vi "Read SVID File.vi"(8 "error in":errorcluster) -> (0 "error out":errorcluster, 3 "SVID Data":T1[](array[typedef]))   [LabVIEW 2020, in "SECS Communication.lvlib" / "SECS Data Class.lvclass"]
uses:
  SECS Data Class.lvclass
  SVID Data.ctl
  SECS-II Class/Format Code.ctl
  <vilib>/DATA AHEAD/XLR8/functions/Workbook/Open Create Workbook XLSX.vi
  <vilib>/DATA AHEAD/XLR8/XLR8.lvlib
  SECS-II Class/SECS-II Class.lvclass
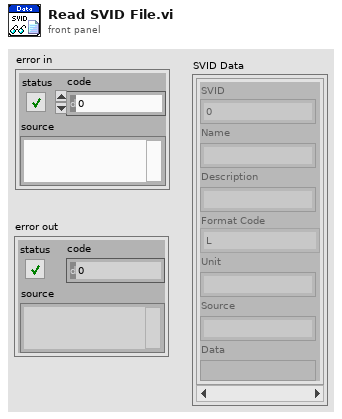
[diagram p1: front panel]
types:
  T1 = typedef "SECS Communication.lvlib/SECS Data Class.lvclass/SVID Data.ctl" = cluster{"SVID":u32, "Name":string, "Description":string, "Format Code":T2, "Unit":string, "Source":string, "Data":variant}
  T2 = typedef "SECS Communication.lvlib/SECS-II Class.lvclass/Format Code.ctl" = enum16{"L", "A", "B", "Boolean", "J", "I1", "I2", "I4", "I8", "U1", "U2", "U4", "U8", "F4", "F8", "Char"}
  T3 = typedef "XLR8.lvlib/XLR8_Ref.ctl" = cluster{"WBK":refnum<k24>, "CurSheet":refnum<k24>, "File":refnum<k24>, "file path":string, "sheet":string, "Sheets":refnum<k24>[], "IsXML":bool, "Policy":i32}
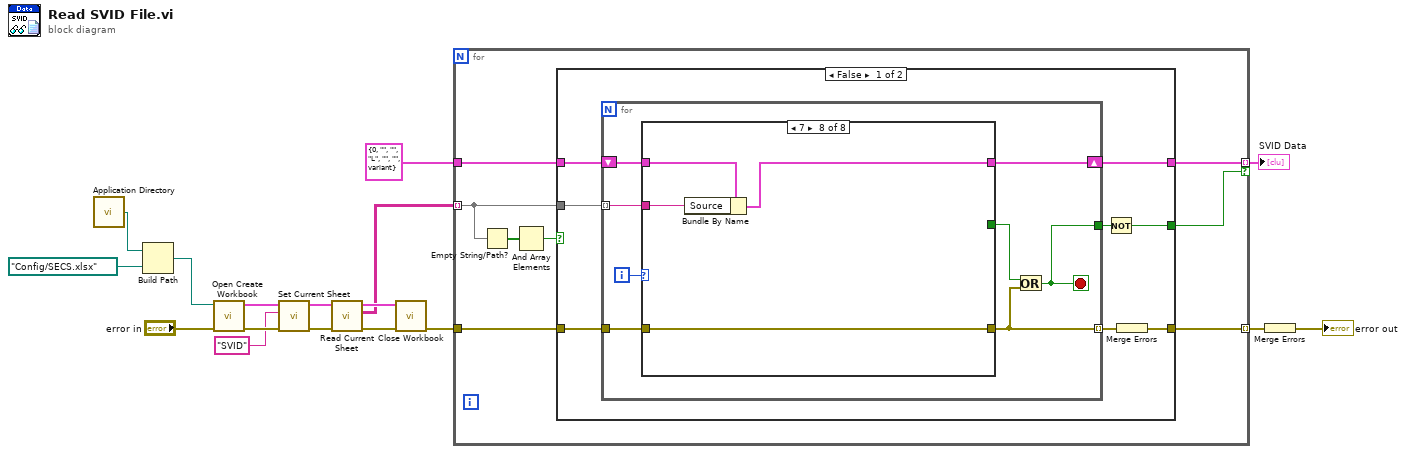
[diagram p0: block diagram]
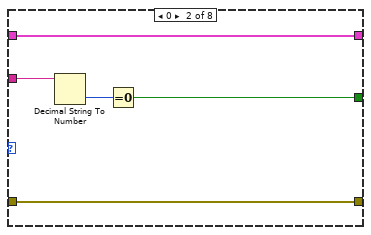
[diagram p3: hidden frame]
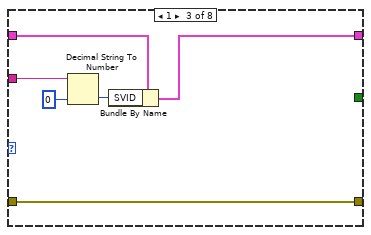
[diagram p4: hidden frame]
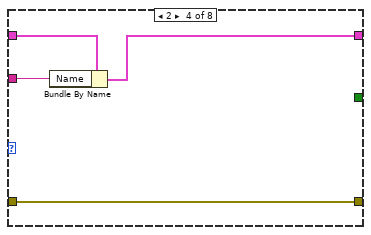
[diagram p5: hidden frame]
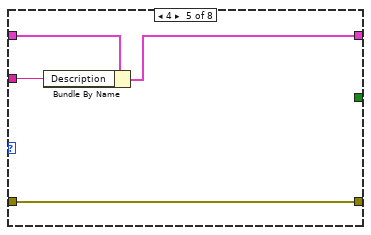
[diagram p6: hidden frame]
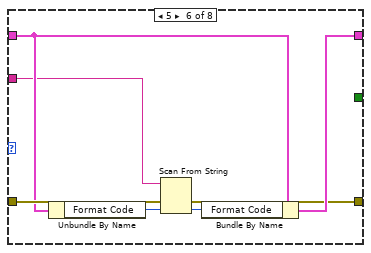
[diagram p7: hidden frame]
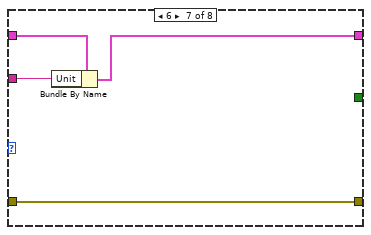
[diagram p8: hidden frame]
diagram:
  n1 = call <vilib>:"Application Directory.vi"() -> ("Application Directory"=w17:path)
  n2 = Build Path(base path=w17, name or relative path=path "Config/SECS.xlsx") -> (appended path=w14:path)
  n3 = call-poly <vilib>:"Open Create Workbook.vi"("error in"="error in", "Workbook Path"=w14) -> ("error out"=w12:errorcluster, "Refs Out"=w13:T3)  [unwired: 8 in]
  n4 = call <vilib>:"Set Current Sheet.vi"("error in"=w12, "Sheet to switch to"="SVID", "Refs In"=w13) -> ("error out"=w9:errorcluster, "Refs Out"=w10:T3)  [unwired: 7 in]
  n5 = call <vilib>:"Read Current Sheet.vi"("error in"=w9, "Refs In"=w10) -> ("error out"=w7:errorcluster, "Sheet-data out"=w5:string[][], "Refs Out"=w8:T3)  [unwired: 7 in]
  n6 = call <vilib>:"Close Workbook.vi"("error in"=w7, "Refs In"=w8) -> ("error out"=w6:errorcluster)  [unwired: 8 in, 1 out]
  n7 = for {
    tunnel: w6 -> [w22]
    tunnel: w5 -> [w23] mode=indexing
    tunnel: T1 {"SVID"=0, "Name"="", "Description"="", "Format Code"=enum."L", "Unit"="", "Source"="", "Data"=variant} ("SVID Data") -> [w21]
    tunnel: [w20] -> w1 mode=indexing if=w19
    tunnel: [w18] -> w3 mode=indexing
    n8 = Empty String/Path?(string/path=w23) -> (empty?=w25:bool[])
    n9 = And Array Elements(Boolean array=w25) -> (logical AND=w24:bool)
    n10 = case shown="False" w24 {
      tunnel: w23 -> [w33 _]
      tunnel: w22 -> [w28 w78]
      tunnel: w21 -> [w32 w79]
      tunnel: [w31 w79] -> w20
      tunnel: [w29 _] -> w19
      tunnel: [w26 w78] -> w18
      frame False {
        n11 = for {
          tunnel: w33 -> [w39] mode=indexing
          shift-right: [w38] -> w31
          shift-left: w32 -> [w41]
          tunnel: [w34] -> w30
          tunnel: w28 -> [w37]
          tunnel: [w35] -> w27 mode=indexing
          i -> [w40]
          stop <- w34 stop-if-true
          n12 = case shown="7" w40 {
            tunnel: w41 -> [w43 w48 w54 w58 w62 w67 w72 w76]
            tunnel: w39 -> [_ w47 w53 w57 w61 w65 w71 w75]
            tunnel: [w43 w48 w50 w56 w60 w69 w73 w77] -> w38
            tunnel: [_ w45 _ _ _ _ _ _] -> w36
            tunnel: w37 -> [w42 w44 w49 w55 w59 w68 w70 w74]
            tunnel: [w42 w44 w49 w55 w59 w63 w70 w74] -> w35
            frame Default {
            }
            frame 0 {
              n13 = Decimal String To Number(string=w47) -> (number=w46:i32)  [unwired: 2 in, 1 out]
              n14 = Equal To 0?(x=w46) -> (x = 0?=w45:bool)
            }
            frame 1 {
              n15 = Decimal String To Number(string=w53, default (0L)=u32 0 ("default (0 I32)")) -> (number=w52:u32)  [unwired: 1 in, 1 out]
              n16 = Bundle By Name(cluster=w54, "SVID"=w52) -> (w50:T1)
            }
            frame 2 {
              n17 = Bundle By Name(cluster=w58, "Name"=w57) -> (w56:T1)
            }
            frame 4 {
              n18 = Bundle By Name(cluster=w62, "Description"=w61) -> (w60:T1)
            }
            frame 5 {
              n19 = Unbundle By Name(w67) -> ("Format Code"=w66:T2)
              n20 = Scan From String(input string=w65, error in=w68, default 1=w66) -> (error out=w63:errorcluster, output 1=w64:T2)  [unwired: 2 in, 2 out]
              n21 = Bundle By Name(cluster=w67, "Format Code"=w64) -> (w69:T1)
            }
            frame 6 {
              n22 = Bundle By Name(cluster=w72, "Unit"=w71) -> (w73:T1)
            }
            frame 7 {
              n23 = Bundle By Name(cluster=w76, "Source"=w75) -> (w77:T1)
            }
          }
          n24 = Or(x=w36, y=w35) -> (x .or. y?=w34:bool)
        }
        n25 = Not(x=w30) -> (.not. x?=w29:bool)
        n26 = Merge Errors(w27) -> (w26:errorcluster)
      }
      frame True {
      }
    }
  }
  "SVID Data" <- w1
  n27 = Merge Errors(w3) -> (→"error out":errorcluster)
